vi "231124_Cluster_MAJ.vi"(8 "error in (no error)":errorcluster, 9 "Nikon status cluster":T1, 10 "Cluster commandes":T2={"Dia lamp"=TRUE, "Dia lamp intensity"=1689.1304347826087, "Objective"=2, "Light path"=2, "Z pos (µm)"=335593} {"Z pos (µm)" min=0 max=990000 step=100 scale=0.0..990000.0; "Light path" items=["1- Eyepiece"=1, "2- Right"=2, "3- Left + Eyepiece"=3, "4- Left"=4]; "Objective" items=["1- Target"=1, "2- PLAN APO 100X 1,45 Oil"=2, "3- Empty"=3, "4- Empty"=4, "5- Empty"=5, "6- Empty"=6]; "Dia lamp intensity" scale=0.0..2100.0}, 11 "Cluster commandes":refnum<vi>) -> (0 "error out":errorcluster, 3 "iLIGHTPATH":i32)   [LabVIEW 2014]
doc: "This vi updates the microscope status cluster.\nThe output is the status of the lightpath (to further display green LEDs accordingly"
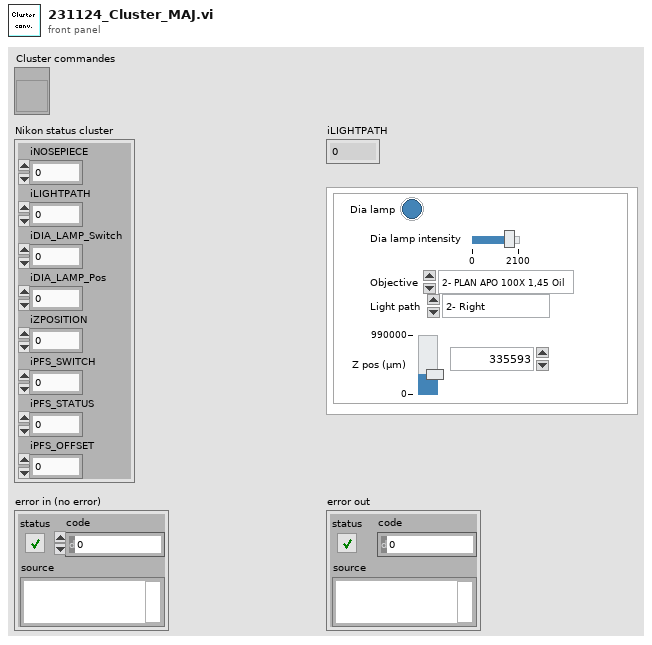
[diagram p1: front panel]
types:
  T1 = cluster{"iNOSEPIECE":i32, "iLIGHTPATH":i32, "iDIA_LAMP_Switch":i32, "iDIA_LAMP_Pos":i32, "iZPOSITION":i32, "iPFS_SWITCH":i32, "iPFS_STATUS":i32, "iPFS_OFFSET":i32}
  T2 = cluster{"Dia lamp":bool, "Dia lamp intensity":dbl, "Objective":i32, "Light path":u32, "Z pos (µm)":i32}
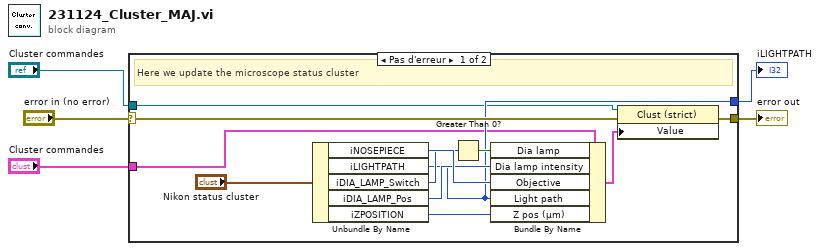
[diagram p0: block diagram]
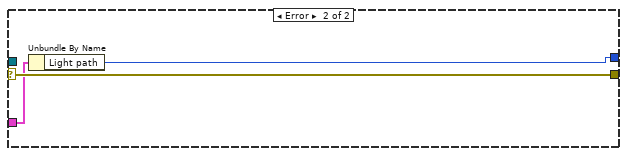
[diagram p2: hidden frame]
diagram:
  n1 = case shown="Pas d'erreur" "error in (no error)" {
    selector: "error in (no error)" -> [w10 w20]
    tunnel: [w11 w20] -> w5
    tunnel: [w9 w18] -> w3
    tunnel: "Cluster commandes" -> [w8 w19]
    tunnel: "Cluster commandes" -> [w6 _]
    frame No Error {
      # "Here we update the microscope status cluster"
      n2 = Unbundle By Name("Nikon status cluster") -> ("iNOSEPIECE"=w16:i32, "iLIGHTPATH"=w9:i32, "iDIA_LAMP_Switch"=w13:i32, "iDIA_LAMP_Pos"=w14:i32, "iZPOSITION"=w17:i32)
      n3 = Greater Than 0?(x=w13) -> (x > 0?=w15:bool)
      n4 = Bundle By Name(cluster=w8, "Dia lamp"=w15, "Dia lamp intensity"=w14, "Objective"=w16, "Light path"=w9, "Z pos (µm)"=w17) -> (w7:T2)
      n5 = property on="Property Node" class="Clust (strict)"(reference=w6, error in=w10, "Value"=w7) -> (error out=w11:errorcluster)  [unwired: 1 out]
    }
    frame Error {
      n6 = Unbundle By Name(w19) -> ("Light path"=w18:u32)
    }
  }
  "error out" <- w5
  "iLIGHTPATH" <- w3
